vi "DiffDrivePoseEst_UpdateWithTime.vi"(4 "RightDistance":dbl, 5 "LeftSpeed":dbl, 6 "LeftDistance":dbl, 7 "RightSpeed":dbl, 9 "GyroAngle":T3={"VALUE"=0.0, "COS"=1.0, "SIN"=0.0} {"SIN" format="%13.4f"; "COS" format="%13.4f"; "VALUE" format="%13.4f"}, 10 "CurrentTimeSeconds":dbl, 11 "in DiffDrivePoseEstimate":T4={"M_VisionContR"=[], "m_nominal_dT"=0.0, "m_PrevTime_Sec"=0.0, "m_GyroOffset"={"VALUE"=0.0, "COS"=1.0, "SIN"=0.0}, "m_PrevAngle"={"VALUE"=0.0, "COS"=1.0, "SIN"=0.0}, "StartLeftEnc_M"=0.0, "StartRightEnc_M"=0.0, "m_Observer"={"m_P"=[], "m_xHat"=[], "States"=0, "Outputs"=0, "m_ContR"=[], "m_ContQ"=[], "m_SigmasF"=[], "m_dT_Sec"=0.0, "MERWE_SCALED_SIGMA_PTS"={"m_Wm"=[], "States"=0, "Alpha"=0.0, "m_Wc"=[], "Kappa"=0}, "meanFuncX"=refnum, "meanFuncY"=refnum, "residualFuncX"=refnum, "residualFuncY"=refnum, "addFuncX"=refnum, "addFuncXExtra"=variant, "residualFuncYExtra"=variant, "residualFuncXExtra"=variant, "MeanFuncYExtra"=variant, "MeanFuncXExtra"=variant, "Inputs"=0}, "m_latencyCompensator"={"m_pastObserverSnapshots "=[]}} {"m_PrevAngle"."SIN" format="%13.4f"; "m_PrevAngle"."COS" format="%13.4f"; "m_PrevAngle"."VALUE" format="%13.4f"; "m_GyroOffset"."SIN" format="%13.4f"; "m_GyroOffset"."COS" format="%13.4f"; "m_GyroOffset"."VALUE" format="%13.4f"}) -> (0 "Error":bool, 2 "Estimated Pose":T1 {"ROTATION"."SIN" format="%13.4f"; "ROTATION"."COS" format="%13.4f"; "ROTATION"."VALUE" format="%13.4f"; "TRANSLATION"."Y" format="%14.3f"; "TRANSLATION"."X" format="%14.3f"}, 3 "Out DiffDrivePoseEstimate":T4={"M_VisionContR"=[], "m_nominal_dT"=0.0, "m_PrevTime_Sec"=0.0, "m_GyroOffset"={"VALUE"=0.0, "COS"=1.0, "SIN"=0.0}, "m_PrevAngle"={"VALUE"=0.0, "COS"=1.0, "SIN"=0.0}, "StartLeftEnc_M"=0.0, "StartRightEnc_M"=0.0, "m_Observer"={"m_P"=[], "m_xHat"=[], "States"=0, "Outputs"=0, "m_ContR"=[], "m_ContQ"=[], "m_SigmasF"=[], "m_dT_Sec"=0.0, "MERWE_SCALED_SIGMA_PTS"={"m_Wm"=[], "States"=0, "Alpha"=0.0, "m_Wc"=[], "Kappa"=0}, "meanFuncX"=refnum, "meanFuncY"=refnum, "residualFuncX"=refnum, "residualFuncY"=refnum, "addFuncX"=refnum, "addFuncXExtra"=variant, "residualFuncYExtra"=variant, "residualFuncXExtra"=variant, "MeanFuncYExtra"=variant, "MeanFuncXExtra"=variant, "Inputs"=0}, "m_latencyCompensator"={"m_pastObserverSnapshots "=[]}} {"m_PrevAngle"."SIN" format="%13.4f"; "m_PrevAngle"."COS" format="%13.4f"; "m_PrevAngle"."VALUE" format="%13.4f"; "m_GyroOffset"."SIN" format="%13.4f"; "m_GyroOffset"."COS" format="%13.4f"; "m_GyroOffset"."VALUE" format="%13.4f"})   [LabVIEW 2019, in "Trajectory_Library.lvlib"]
doc: "Updates the the Unscented Kalman Filter using only wheel encoder information. Note that this should be called every loop.\n\nInputs:\n - LeftSpeed -- Left wheel speed (meters/sec)\n - RightSpeed -- Right wheel speed (meters/sec)\n - inDiffDrivePoseEst -- system data cluster\n - gyroAngle -- The current gyro angle. (radians)\n - currentTime -- Time at which this method was called, in seconds.\n - distanceLeftMeters -- The total distance travelled by the left wheel in meters. This can be the encoder reading.\n - distanceRightMeters -- The total distance travelled by the right wheel in meters. This can be the encoder reading.\n\nOutputs:\n - outDiffDrivePoseEst -- system data cluster\n - EstimatedPose -- The estimated pose of the robot in meters."
uses:
  Trajectory_Library.lvlib
  <vilib>/Analysis/Matrix/Datatypes/RealMatrix.ctl
  <vilib>/Analysis/Matrix/NI_Matrix.lvlib
  MERWE_SCALED_SIGMA_PTS.ctl
  UNSCENTED_KALMAN_FILTER.ctl
  CALLBACK_FUNC_TYPE.ctl
  OBSERVER_SNAPSHOT.ctl
  OBSERVER_SNAP_LIST_ITEM.ctl
  KALMAN_FILTER_LATENCY_COMP.ctl
  DIFF_DRIVE_POSE_EST.ctl
  ROTATION2D.ctl
  TRANSLATION2D.ctl
  POSE2D.ctl
panel:
  # "<3, 3>"
  # "<Statess,1>"
  # "<States, States>"
  # "<Inputs, 1>"
  # "<Outputs,  1>"
  # "State Estimate <Statess,1>"
  # "<States, States>"
  # "<States, ?>"
  # "<Statess,  States>"
  # "<Outputs, Outputs>"
  # "<?, 1>"
  # "<?, 1>"
  # "<3, 3>"
  # "<Statess,1>"
  # "<States, States>"
  # "<Inputs, 1>"
  # "<Outputs,  1>"
  # "State Estimate <Statess,1>"
  # "<States, States>"
  # "<States, ?>"
  # "<Statess,  States>"
  # "<Outputs, Outputs>"
  # "<?, 1>"
  # "<?, 1>"
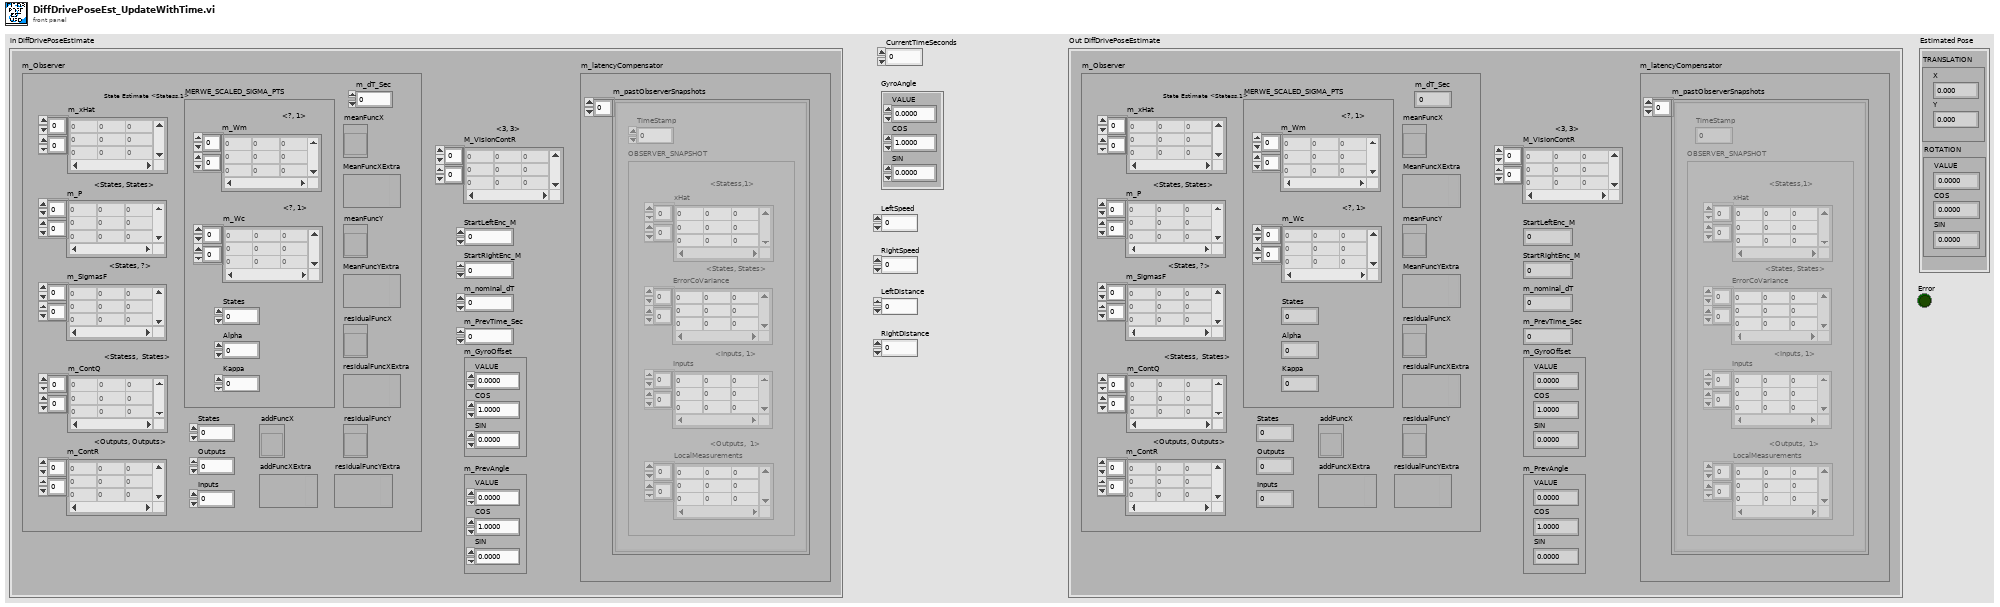
[diagram p1: front panel]
types:
  T1 = typedef "Trajectory_Library.lvlib/POSE2D.ctl" = cluster{"TRANSLATION":T2, "ROTATION":T3}
  T2 = typedef "Trajectory_Library.lvlib/TRANSLATION2D.ctl" = cluster{"X":dbl, "Y":dbl}
  T3 = typedef "Trajectory_Library.lvlib/ROTATION2D.ctl" = cluster{"VALUE":dbl, "COS":dbl, "SIN":dbl}
  T4 = typedef "Trajectory_Library.lvlib/DIFF_DRIVE_POSE_EST.ctl" = cluster{"M_VisionContR":T5, "m_nominal_dT":dbl, "m_PrevTime_Sec":dbl, "m_GyroOffset":T3, "m_PrevAngle":T3, "StartLeftEnc_M":dbl, "StartRightEnc_M":dbl, "m_Observer":T6, "m_latencyCompensator":T9}
  T5 = typedef "NI_Matrix.lvlib/RealMatrix.ctl" = dbl[][]
  T6 = typedef "Trajectory_Library.lvlib/UNSCENTED_KALMAN_FILTER.ctl" = cluster{"m_P":T5, "m_xHat":T5, "States":i32, "Outputs":i32, "m_ContR":T5, "m_ContQ":T5, "m_SigmasF":T5, "m_dT_Sec":dbl, "MERWE_SCALED_SIGMA_PTS":T7, "meanFuncX":T8, "meanFuncY":T8, "residualFuncX":T8, "residualFuncY":T8, "addFuncX":T8, "addFuncXExtra":variant, "residualFuncYExtra":variant, "residualFuncXExtra":variant, "MeanFuncYExtra":variant, "MeanFuncXExtra":variant, "Inputs":i32}
  T7 = typedef "Trajectory_Library.lvlib/MERWE_SCALED_SIGMA_PTS.ctl" = cluster{"m_Wm":T5, "States":i32, "Alpha":dbl, "m_Wc":T5, "Kappa":i32}
  T8 = typedef "Trajectory_Library.lvlib/CALLBACK_FUNC_TYPE.ctl" = refnum<vi>
  T9 = typedef "Trajectory_Library.lvlib/KALMAN_FILTER_LATENCY_COMP.ctl" = cluster{"m_pastObserverSnapshots ":T10[]}
  T10 = typedef "Trajectory_Library.lvlib/OBSERVER_SNAP_LIST_ITEM.ctl" = cluster{"TimeStamp":dbl, "OBSERVER_SNAPSHOT":T11}
  T11 = typedef "Trajectory_Library.lvlib/OBSERVER_SNAPSHOT.ctl" = cluster{"ErrorCoVariance":T5, "xHat":T5, "LocalMeasurements":T5, "Inputs":T5}
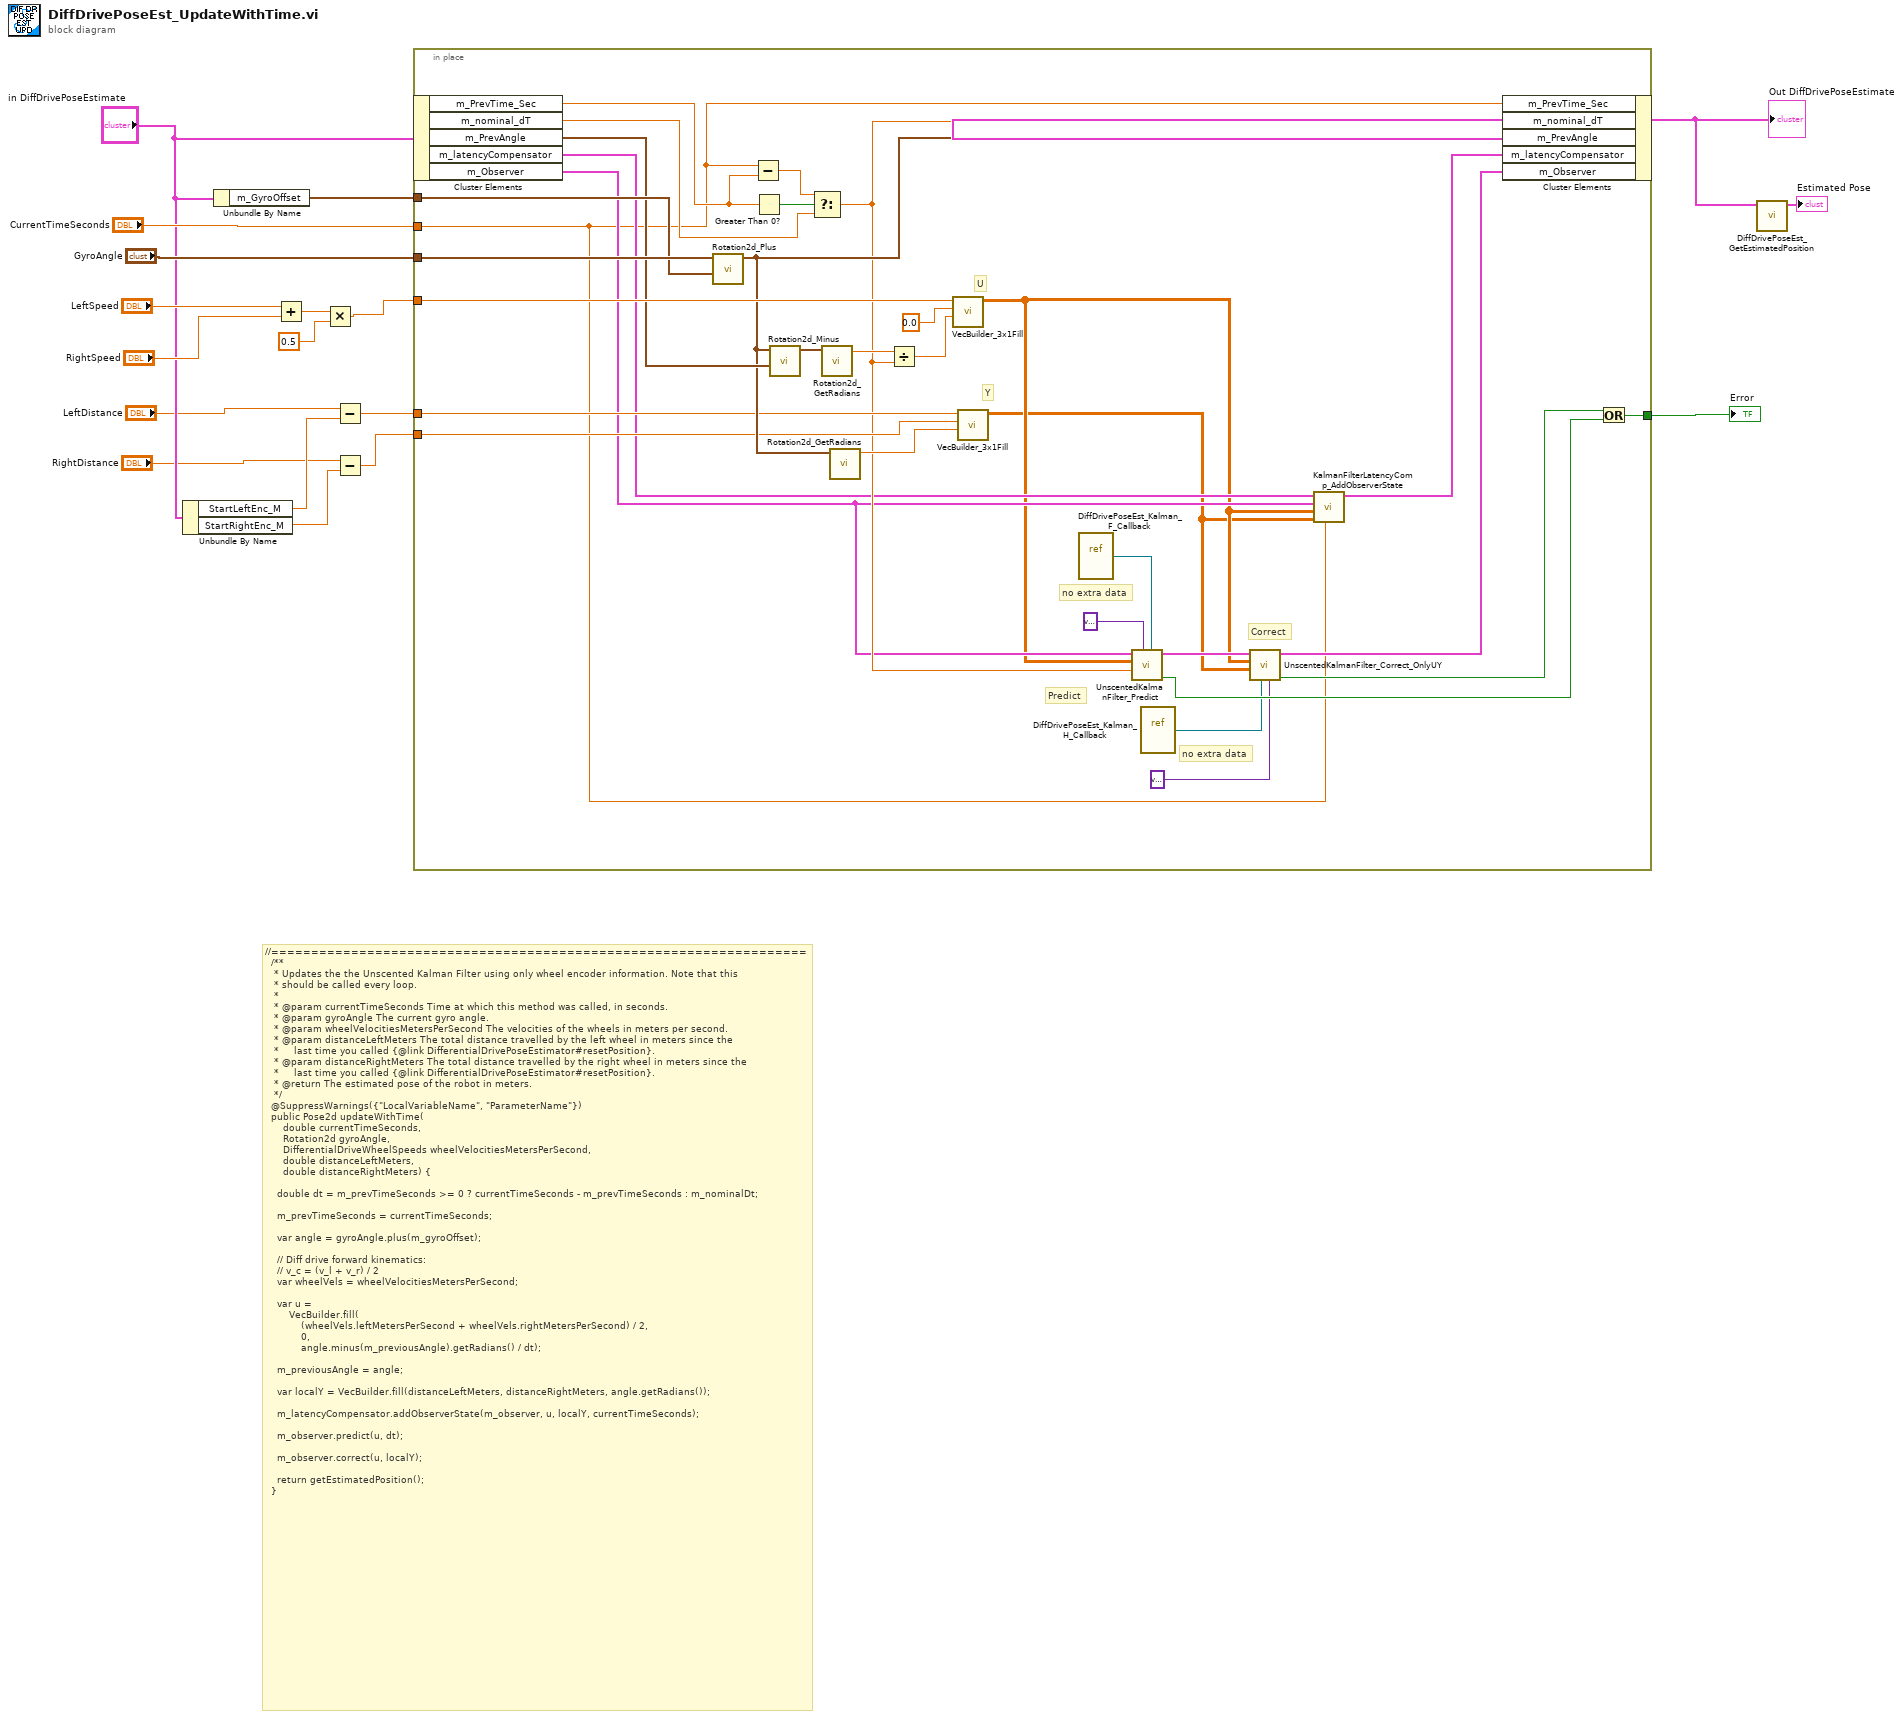
[diagram p0: block diagram]
diagram:
  # "//===================================================================\n  /**\n   * Updates the the Unscented Kalman Filter using only wheel encoder information. Note that this\n   * should be called every loop.\n   *\n   * @param currentTimeSeconds Time at which this method was called, in seconds.\n   * @param gyroAngle The current gyro angle.\n   * @param wheelVelocitiesMetersPerSecond The velocities of the wheels in meters per second.\n   * @param distanceLeftMeters The total distance travelled by the left wheel in meters since the\n   *     last time you called {@link DifferentialDrivePoseEstimator#resetPosition}.\n   * @param distanceRightMeters The total distance travelled by the right wheel in meters since the\n   *     last time you called {@link DifferentialDrivePoseEstimator#resetPosition}.\n   * @return The estimated pose of the robot in meters.\n   */\n  @SuppressWarnings({\"LocalVariableName\", \"ParameterName\"})\n  public Pose2d updateWithTime(\n      double currentTimeSeconds,\n      Rotation2d gyroAngle,\n      DifferentialDriveWheelSpeeds wheelVelocitiesMetersPerSecond,\n      double distanceLeftMeters,\n      double distanceRightMeters) {\n\n    double dt = m_prevTimeSeconds >= 0 ? currentTimeSeconds - m_prevTimeSeconds : m_nominalDt;\n\n    m_prevTimeSeconds = currentTimeSeconds;\n\n    var angle = gyroAngle.plus(m_gyroOffset);\n\n    // Diff drive forward kinematics:\n    // v_c = (v_l + v_r) / 2\n    var wheelVels = wheelVelocitiesMetersPerSecond;\n\n    var u =\n        VecBuilder.fill(\n            (wheelVels.leftMetersPerSecond + wheelVels.rightMetersPerSecond) / 2,\n            0,\n            angle.minus(m_previousAngle).getRadians() / dt);\n\n    m_previousAngle = angle;\n\n    var localY = VecBuilder.fill(distanceLeftMeters, distanceRightMeters, angle.getRadians());\n\n    m_latencyCompensator.addObserverState(m_observer, u, localY, currentTimeSeconds);\n\n    m_observer.predict(u, dt);\n\n    m_observer.correct(u, localY);\n\n    return getEstimatedPosition();\n  }"
  n1 = Unbundle By Name("in DiffDrivePoseEstimate") -> ("StartLeftEnc_M"=w4:dbl, "StartRightEnc_M"=w3:dbl)
  n2 = Unbundle By Name("in DiffDrivePoseEstimate") -> ("m_GyroOffset"=w11:T3)
  n3 = Add(x="LeftSpeed", y="RightSpeed") -> (x+y=w14:dbl)
  n4 = Multiply(x=w14, y=0.5) -> (x*y=w12:dbl)
  n5 = Subtract(x="LeftDistance", y=w4) -> (x-y=w6:dbl)
  n6 = Subtract(x="RightDistance", y=w3) -> (x-y=w5:dbl)
  n7 = in-place {
    in-place-border: "CurrentTimeSeconds" -> [w19]
    in-place-border: "GyroAngle" -> [w47]
    in-place-border: w12 -> [w46]
    in-place-border: w11 -> [w44]
    in-place-border: w6 -> [w37]
    in-place-border: w5 -> [w36]
    in-place-border: [w31] -> w8
    # "Correct"
    # "Predict"
    # "no extra data"
    # "no extra data"
    # "Y"
    # "U"
    n8 = in-place-cluster #1("in DiffDrivePoseEstimate") -> ("m_PrevTime_Sec"=w49:dbl, "m_nominal_dT"=w41:dbl, "m_PrevAngle"=w43:T3, "m_latencyCompensator"=w23:T9, "m_Observer"=w22:T6)
    n9 = call "Rotation2d_Plus.vi"("other ROTATION"=w44, "in ROTATION"=w47) -> ("out ROTATION"=w38:T3)  [unwired: 9 in]
    n10 = Subtract(x=w19, y=w49) -> (x-y=w48:dbl)
    n11 = Greater Than 0?(x=w49) -> (x > 0?=w50:bool)
    n12 = call "Rotation2d_Minus.vi"("other ROTATION"=w43, "in ROTATION"=w38) -> ("out ROTATION"=w42:T3)  [unwired: 9 in]
    n13 = Select(t=w48, s=w50, f=w41) -> (s? t:f=w30:dbl)
    n14 = call "Rotation2d_GetRadians.vi"("in ROTATION"=w42) -> ("AngleRadians"=w40:dbl)  [unwired: 10 in]
    n15 = call "Rotation2d_GetRadians.vi"("in ROTATION"=w38) -> ("AngleRadians"=w35:dbl)  [unwired: 10 in]
    n16 = Divide(x=w40, y=w30) -> (x/y=w39:dbl)
    n17 = call "VecBuilder_3x1Fill.vi"("R2"=w39, "R1"=0.0, "R0"=w46) -> ("output matrix"=w21:T5)  [unwired: 8 in]
    n18 = call "VecBuilder_3x1Fill.vi"("R2"=w35, "R1"=w36, "R0"=w37) -> ("output matrix"=w20:T5)  [unwired: 8 in]
    n19 = vi-ref "DiffDrivePoseEst_Kalman_F_Callback.vi"() -> (w29:refnum<vi>)
    n20 = call "UnscentedKalmanFilter_Predict.vi"("f_Func"=w29, "F_Func_ExtraData"=variant, "dT_Seconds"=w30, "U"=w21, "in UnscentedKalmanFiilter"=w22) -> ("Error"=w32:bool, "out UnscentedKalmanFiilter"=w34:T6)  [unwired: 5 in]
    n21 = vi-ref "DiffDrivePoseEst_Kalman_H_Callback.vi"() -> (w27:refnum<vi>)
    n22 = call "UnscentedKalmanFilter_Correct_OnlyUY.vi"("H_ExtraData"=variant ("F_Func_ExtraData"), "H_Func"=w27, "Y"=w20, "U"=w21, "in UnscentedKalmanFiilter"=w34) -> ("Error"=w33:bool, "out UnscentedKalmanFiilter"=w25:T6)  [unwired: 5 in]
    n23 = call "KalmanFilterLatencyComp_AddObserverState.vi"("TimeStamp_Sec"=w19, "Local Y"=w20, "U"=w21, "Observer"=w22, "in KalmanFilterLatencyCompensator"=w23) -> ("out KalmanFilterLatencyCompensator"=w24:T9)  [unwired: 6 in]
    n24 = in-place-cluster #1("m_PrevTime_Sec"=w19, "m_nominal_dT"=w30, "m_PrevAngle"=w38, "m_latencyCompensator"=w24, "m_Observer"=w25) -> (w10:T4)
    n25 = Or(x=w33, y=w32) -> (x .or. y?=w31:bool)
  }
  "Out DiffDrivePoseEstimate" <- w10
  "Error" <- w8
  n26 = call "DiffDrivePoseEst_GetEstimatedPosition.vi"("in DiffDrivePoseEstimate"=w10) -> ("Estimated Pose"=→"Estimated Pose":T1)  [unwired: 10 in]
